vi "mono_send_command.vi"(3 "error in (no error)":errorcluster, 4 "JSON Command":string, 5 "TCP Network Connection in":refnum<k5>) -> (0 "error out":errorcluster, 2 "response":string)   [LabVIEW 2018, in "monoDrive.lvlib"]
uses:
  monoDrive.lvlib
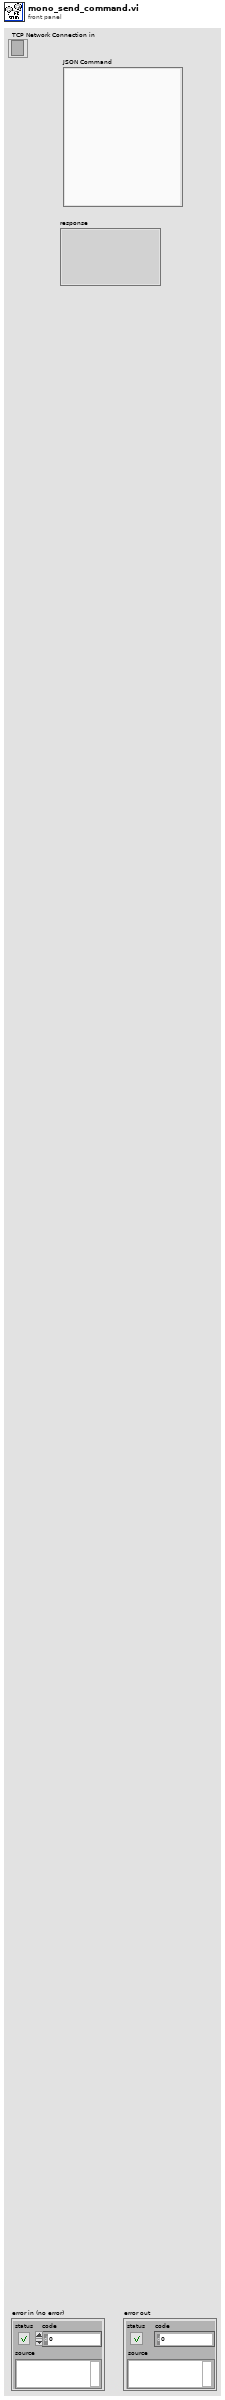
[diagram p1: front panel]
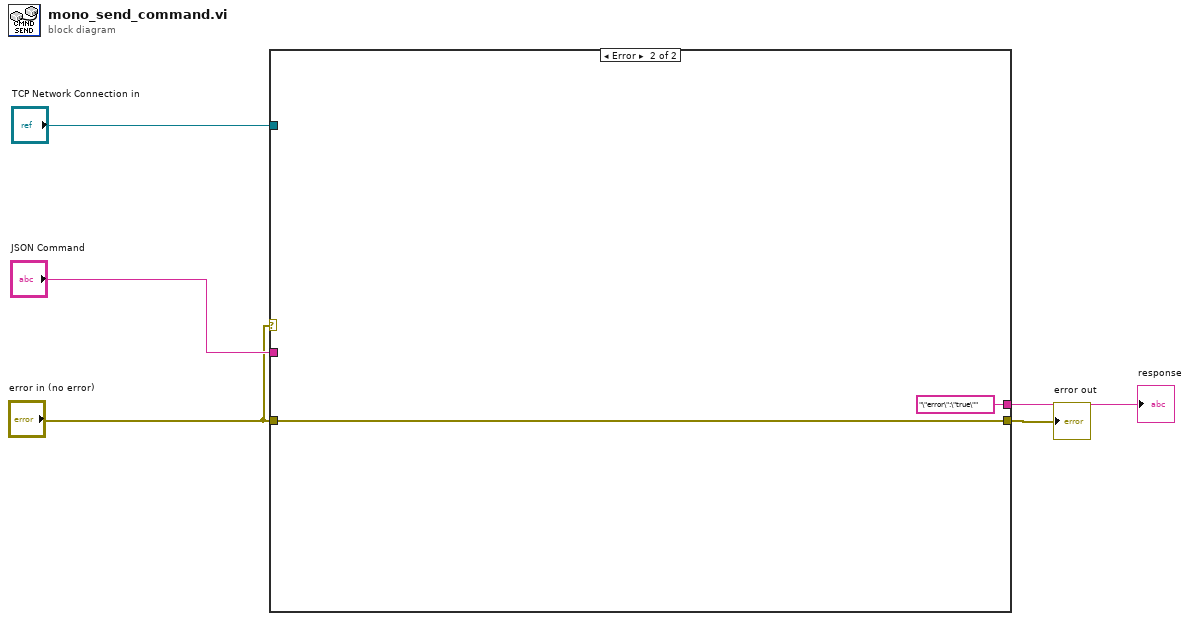
[diagram p0: block diagram]
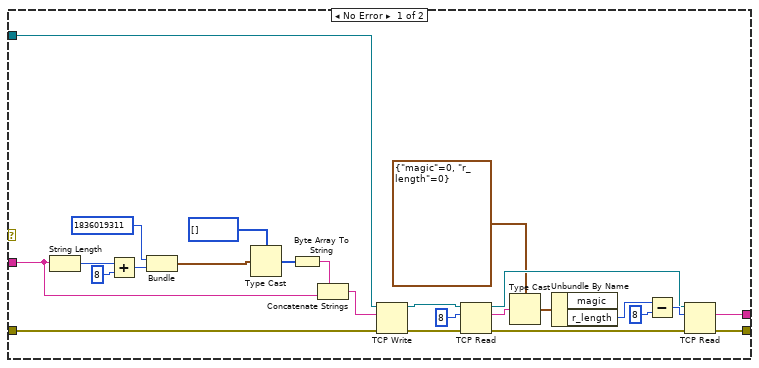
[diagram p2: hidden frame]
diagram:
  n1 = case shown="Error" "error in (no error)" {
    tunnel: [w30 w32] -> w5
    tunnel: [w10 "\"error\":\"true\"" ("data out")] -> w4
    tunnel: "error in (no error)" -> [w9 w32]
    tunnel: "TCP Network Connection in" -> [w8 _]
    tunnel: "JSON Command" -> [w7 _]
    frame No Error {
      n2 = String Length(string=w7) -> (length=w11:i32)
      n3 = Add(x=w11, y=u32 8) -> (x+y=w22:u32)
      n4 = Bundle(u32 1836019311, w22) -> (w27:cluster{u32, u32})  [unwired: 1 in]
      n5 = Type Cast(type=u8[] [], x=w27) -> (*(type *) &x=w25:u8[])
      n6 = Byte Array To String(unsigned byte array=w25) -> (string=w21:string)
      n7 = Concatenate Strings(w21, w7) -> (w6:string)
      n8 = TCP Write(connection ID=w8, data in=w6, error in (no error)=w9) -> (connection ID out=w28:refnum<k5>, error out=w29:errorcluster)  [unwired: 1 in, 1 out]
      n9 = TCP Read(connection ID=w28, bytes to read=8, error in (no error)=w29) -> (connection ID out=w15:refnum<k5>, data out=w20:string, error out=w16:errorcluster)  [unwired: 2 in]
      n10 = Type Cast(type=cluster{"magic":u32, "r_length":u32} {"magic"=0, "r_length"=0}, x=w20) -> (*(type *) &x=w19:cluster{"magic":u32, "r_length":u32})
      n11 = Unbundle By Name(w19) -> ("r_length"=w17:u32)  [unwired: 1 out]
      n12 = Subtract(x=w17, y=u32 8) -> (x-y=w18:u32)
      n13 = TCP Read(connection ID=w15, bytes to read=w18, error in (no error)=w16) -> (data out=w10:string, error out=w30:errorcluster)  [unwired: 2 in, 1 out]
    }
    frame Error {
    }
  }
  "error out" <- w5
  "response" <- w4
